vi "Pre Launch Init.vi"(8 "error in (no error)":errorcluster) -> (0 "error out":errorcluster, 3 "Event Registration Refnum":refnum<event-registration>)   [LabVIEW 2021, in "Error Handling.lvlib"]
uses:
  Error Handling.lvlib
  User Event/UE Dataset.ctl
  Private Controls/Q Control.ctl
  User Event/UE Control.ctl
  User Event/User Event.lvlib
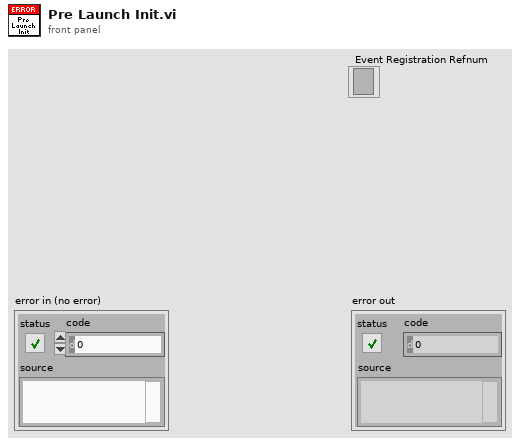
[diagram p1: front panel]
types:
  T1 = typedef "User Event.lvlib/UE Control.ctl" = enum16{"Create", "Get", "Generate", "Destroy"}
  T2 = typedef "Error Handling.lvlib/Q Control.ctl" = enum16{"Obtain", "Get", "Release"}
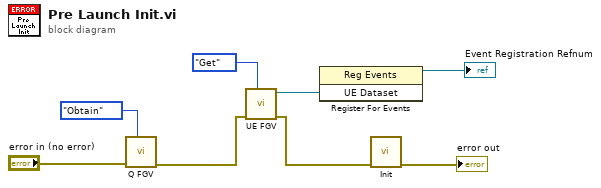
[diagram p0: block diagram]
diagram:
  n1 = call "Q FGV.vi"("Q Control"=Q_Control."Obtain", "error in (no error)"="error in (no error)") -> ("error out"=w4:errorcluster)  [unwired: 8 in, 1 out]
  n2 = call "UE FGV.vi"("UE Ctls"=UE_Control."Get", "error in (no error)"=w4) -> ("error out"=w3:errorcluster, "UE Dataset"=w1:refnum<user-event>)  [unwired: 8 in]
  n3 = register-events(w1) -> (reference out=→"Event Registration Refnum":refnum<event-registration>)  [unwired: 2 in, 1 out]
  n4 = call "Init.vi"("error in (no error)"=w3) -> ("error out"=→"error out":errorcluster)  [unwired: 10 in]
